vi "Initialize controls.vi"(8 "error in (no error)":errorcluster, 11 "Cluster":T1) -> (0 "error out":errorcluster)   [LabVIEW 2017]
uses:
  Controls/Testscreen_Input cluster.ctl
  <vilib>/addons/database/Connection.llb/Conn ObjectReference.ctl
  <vilib>/addons/database/NI_Database_API.lvlib
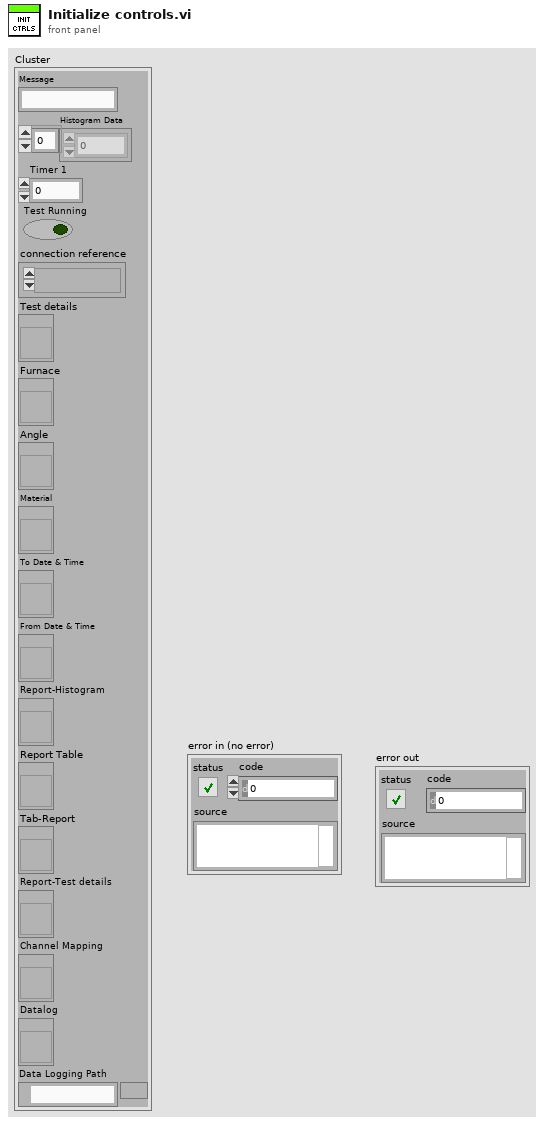
[diagram p1: front panel]
types:
  T1 = typedef "Testscreen_Input cluster.ctl" = cluster{"Message":string, "Histogram Data":i32[], "Timer 1":u32, "Test Running":bool, "connection reference":T2, "Test details":refnum<vi>, "Furnace":refnum<vi>, "Angle":refnum<vi>, "Material":refnum<vi>, "To Date & Time":refnum<vi>, "From Date & Time":refnum<vi>, "Report-Histogram":refnum<vi>, "Report Table":refnum<vi>, "Tab-Report":refnum<vi>, "Report-Test details":refnum<vi>, "Channel Mapping":refnum<vi>, "Datalog":refnum<vi>, "Data Logging Path":path}
  T2 = typedef "NI_Database_API.lvlib/Conn ObjectReference.ctl" = refnum<k1>
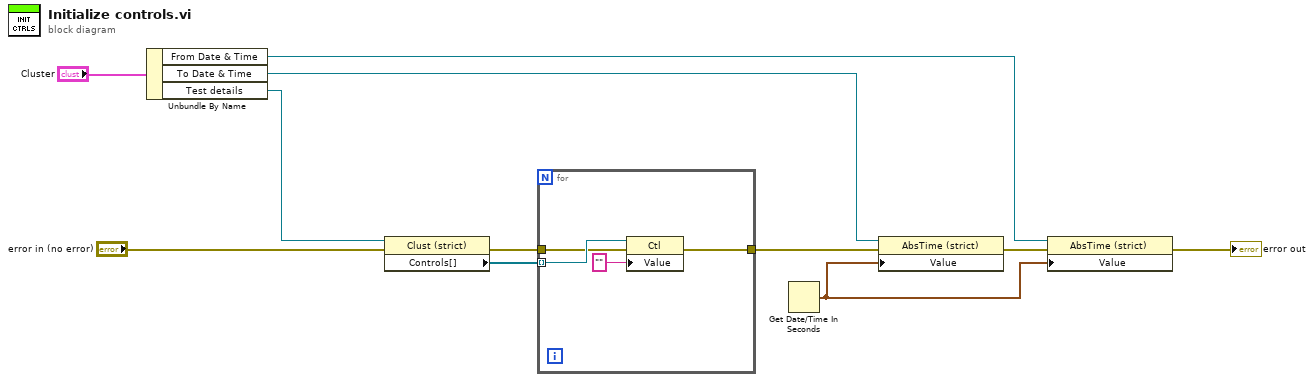
[diagram p0: block diagram]
diagram:
  n1 = Unbundle By Name("Cluster") -> ("From Date & Time"=w5:refnum<vi>, "To Date & Time"=w6:refnum<vi>, "Test details"=w10:refnum<vi>)
  n2 = property class="Clust (strict)"(reference=w10, error in="error in (no error)") -> (error out=w7:errorcluster, "Controls[]"=w8:refnum<vi>[])  [unwired: 1 out]
  n3 = for {
    tunnel: w8 -> [w15] mode=indexing
    tunnel: [w13] -> w3
    tunnel: w7 -> [w12]
    n4 = property class="Ctl"(reference=w15, error in=w12, "Value"="") -> (error out=w13:errorcluster)  [unwired: 1 out]
  }
  n5 = Get Date/Time In Seconds() -> (seconds since 1Jan1904=w1:timestamp)
  n6 = property class="AbsTime (strict)"(reference=w6, error in=w3, "Value"=w1) -> (error out=w4:errorcluster)  [unwired: 1 out]
  n7 = property class="AbsTime (strict)"(reference=w5, error in=w4, "Value"=w1) -> (error out=→"error out":errorcluster)  [unwired: 1 out]
